vi "Voltage (with Events) - Continuous Input.vi"() -> ()   [LabVIEW 2022 SP3]
doc: "This example demonstrates how to continuously acquire buffered voltage measurements using a DAQmx device. It uses software events to ensure that the program does not become unresponsive while waiting for samples to become available.\n\nFor instructions on how to connect your signals to the DAQ device, refer to your device documentation."
uses:
  <vilib>/Utility/error.llb/DialogType.ctl
  <vilib>/DAQmx/read.llb/DAQmx Read (Analog 1D Wfm NChan NSamp).vi
  <vilib>/DAQmx/create/channels.llb/DAQmx Create Channel (AI-Voltage-Basic).vi
  <vilib>/DAQmx/configure/timing.llb/DAQmx Timing (Sample Clock).vi
  <vilib>/DAQmx/configure/task.llb/DAQmx Configure Logging (TDMS).vi
  <vilib>/DAQmx/configure/trigger.llb/DAQmx Start Trigger (Digital Edge).vi
  <vilib>/DAQmx/configure/trigger.llb/DAQmx Start Trigger (Time).vi
  <vilib>/DAQmx/configure/trigger.llb/DAQmx Start Trigger (Analog Edge).vi
  <vilib>/DAQmx/miscellaneous.llb/DAQmx Fill In Error Info.vi
  <resource>/objmgr/daqmx.rc
panel:
  in  "Trigger Type":T1(tab)
  in  "Digital Start Trigger Edge":i32(ring)=10280 caption="Edge" items=["Rising"=10280, "Falling"=10171]
  in  "Digital Start Trigger Source":tag="/Dev1/PFI0" caption="Source"
  in  "Digital Pause Trigger Pause When":i32(ring)=10192 caption="Pause When" items=["High"=10192, "Low"=10214]
  in  "Digital Pause Trigger Source":tag="/Dev1/PFI0" caption="Source"
  in  "Analog Start Trigger Level":dbl caption="Level" format="%0.2f"
  in  "Analog Start Trigger Hysteresis":dbl caption="Hysteresis" format="%.2f"
  in  "Analog Start Trigger Slope":i32(ring)=10280 caption="Slope" items=["Rising"=10280, "Falling"=10171]
  in  "Analog Start Trigger Source":string="APFI0" caption="Source"
  in  "Analog Pause Trigger Source":string="APFI0" caption="Source"
  in  "Analog Pause Trigger Pause When":i32(ring)=10093 caption="Pause When" items=["Above Level"=10093, "Below Level"=10107]
  in  "Analog Pause Trigger Level":dbl caption="Level" format="%.2f"
  in  "When":timestamp
  in  "Select Time\nManually":bool
  in  "Stop":bool
  out "Waveform Graph":waveform(dbl)[](graph)
  in  "TDMS File Path":path
  in  "Samples per Loop":i32=100
  in  "Sample Rate":dbl=1000.0
  in  "Sample Clock Source":tag="OnboardClock"
  in  "Terminal Configuration":i32(ring)=-1 items=["default"=-1, "RSE"=10083, "NRSE"=10078, "Differential"=10106, "Pseudodifferential"=12529]
  in  "Max Voltage":dbl=5.0
  in  "Min Voltage":dbl=-5.0
  in  "Physical Channel":tag="Dev1/ai0"
  out "Actual Sample Rate":dbl format="%0.2f"
  in  "Logging Mode":i32(ring)=10231 items=["Off"=10231, "Log and Read"=15842]
  # "Channel Settings"
  # "Acquired Data"
  # "Timing Settings"
  # "Trigger Settings"
  # "Logging Settings"
  # "To enable triggers, select a tab above, and configure the settings.\n\nNot all hardware supports all trigger types. Refer to your device documentation for more information."
  # "This trigger type is not supported in continuous sample timing. \n\nRefer to your device documentation for more information on which triggers are supported."
  # "This trigger type is not supported in continuous sample timing. \n\nRefer to your device documentation for more information on which triggers are supported."
  # "If time is not manually set, task will begin after 10 seconds"
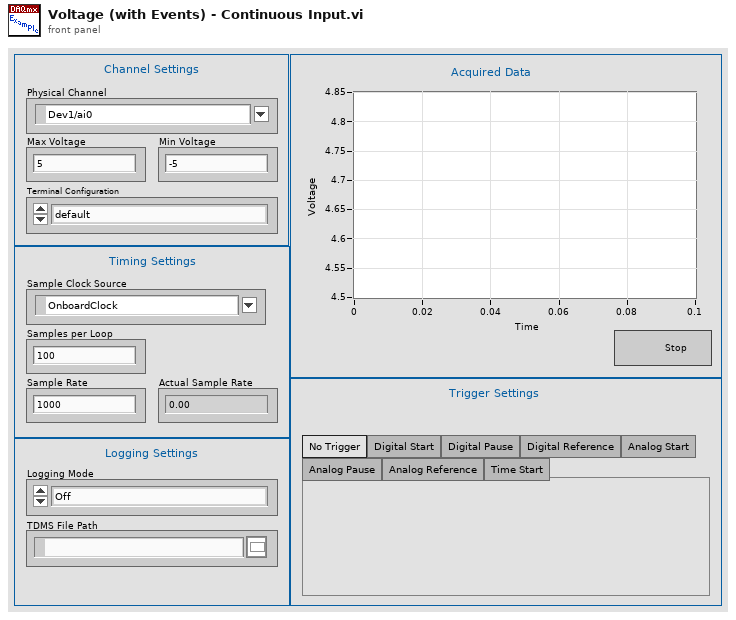
[diagram p1: front panel]
types:
  T1 = enum32{"No Trigger", "Digital Start", "Digital Pause", "Digital Reference", "Analog Start", "Analog Pause", "Analog Reference", "Time Start"}
  T2 = typedef "DialogType.ctl" = u16
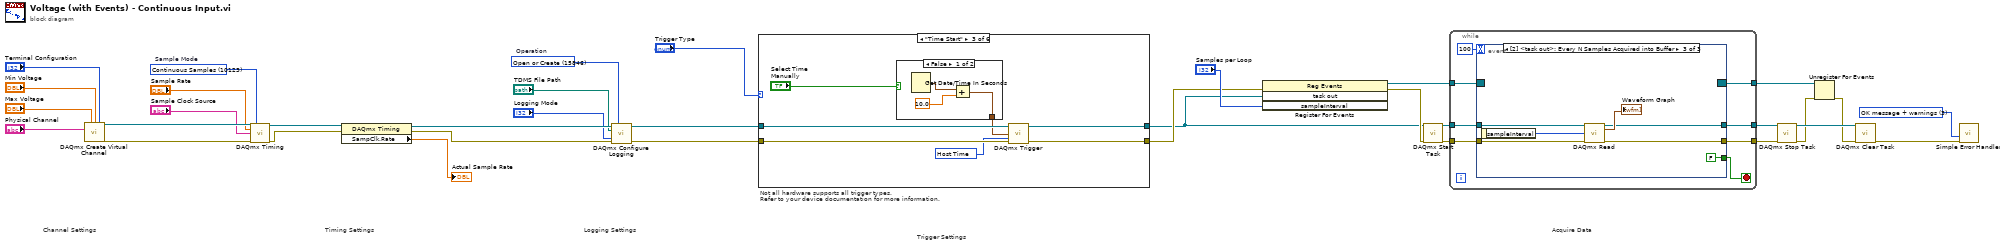
[diagram p0: block diagram]
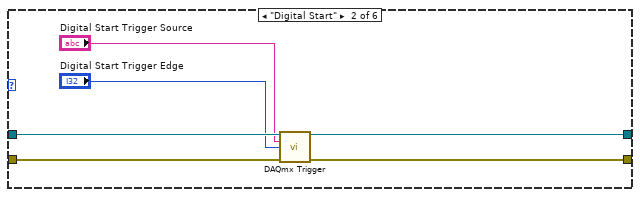
[diagram p3: hidden frame]
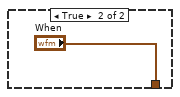
[diagram p4: hidden frame]
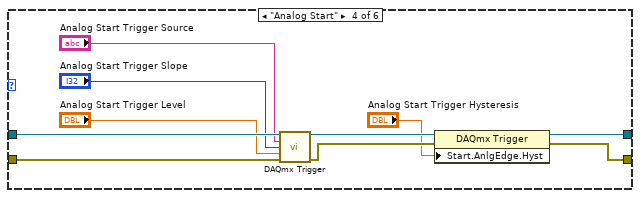
[diagram p5: hidden frame]
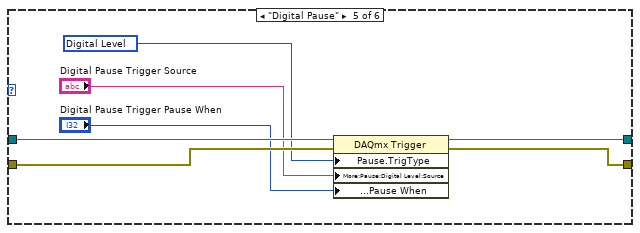
[diagram p6: hidden frame]
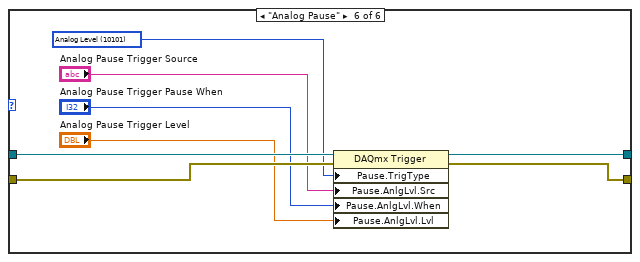
[diagram p7: hidden frame]
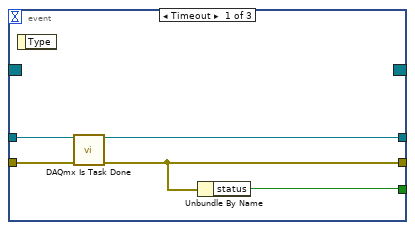
[diagram p8: hidden frame]
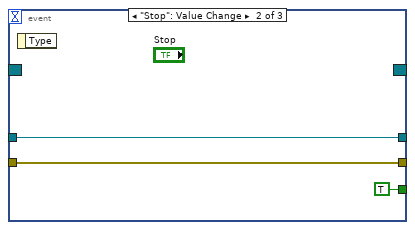
[diagram p9: hidden frame]
diagram:
  w9 = T2 3 items=["no dialog", "OK message", "continue or stop message", "OK message + warnings", "continue/stop + warnings"] ("type of dialog (OK msg:1)")
  w28 = 15846 items=["Open"=10437, "Open or Create"=15846, "Create or Replace"=15847, "Create"=15848]  # Operation
  w33 = 10123 items=["Finite Samples"=10178, "Continuous Samples"=10123, "Hardware Timed Single Point"=12522]  # Sample Mode
  # "Trigger Settings"
  # "Not all hardware supports all trigger types.\nRefer to your device documentation for more information."
  # "Acquire Data"
  # "Logging Settings"
  # "Timing Settings"
  # "Channel Settings"
  n1 = call-poly <vilib>:"DAQmx Create Virtual Channel.vi"("maximum value"="Max Voltage", "minimum value"="Min Voltage", "input terminal configuration"="Terminal Configuration", "physical channels"="Physical Channel") -> ("task out"=w31:refnum<k21>, "error out"=w32:errorcluster)  [unwired: 10 in]
  n2 = call-poly <vilib>:"DAQmx Timing.vi"("task/channels in"=w31, "sample mode"=w33, "rate"="Sample Rate", "source"="Sample Clock Source", "error in"=w32) -> ("task out"=w35:refnum<k21>, "error out"=w34:errorcluster)  [unwired: 9 in]
  n3 = property class="DAQmx Timing"(reference=w35, error in=w34) -> (reference out=w30:refnum<k21>, error out=w29:errorcluster, "SampClk.Rate"=→"Actual Sample Rate":dbl)
  n4 = call-poly <vilib>:"DAQmx Configure Logging.vi"("task/channels in"=w30, "operation"=w28, "file path"="TDMS File Path", "logging mode"="Logging Mode", "error in"=w29) -> ("task out"=w2:refnum<k21>, "error out"=w1:errorcluster)  [unwired: 9 in]
  n5 = case shown="\"Time Start\"" "Trigger Type" {
    tunnel: w2 -> [w37 w43 w50 w64 w71 w79]
    tunnel: w1 -> [w36 w42 w49 w63 w68 w76]
    tunnel: [w37 w41 w48 w61 w70 w78] -> w3
    tunnel: [w36 w40 w47 w60 w69 w77] -> w4
    frame "No Trigger", Default {
    }
    frame "Digital Start" {
      n6 = call-poly <vilib>:"DAQmx Trigger.vi"("task/channels in"=w43, "source"="Digital Start Trigger Source", "edge"="Digital Start Trigger Edge", "error in"=w42) -> ("task out"=w41:refnum<k21>, "error out"=w40:errorcluster)  [unwired: 10 in]
    }
    frame "Time Start" {
      w46 = 16126 items=["Host Time"=16126, "I/O Device Time"=16127] ("timescale")
      n7 = case shown="False" "Select Time\nManually" {
        tunnel: [w52 "When"] -> w44
        frame False {
          n8 = Get Date/Time In Seconds() -> (seconds since 1Jan1904=w53:timestamp)
          n9 = Add(x=w53, y=10.0) -> (x+y=w52:timestamp)
        }
        frame True {
        }
      }
      n10 = call-poly <vilib>:"DAQmx Trigger.vi"("task/channels in"=w50, "when"=w44, "timescale"=w46, "error in"=w49) -> ("task out"=w48:refnum<k21>, "error out"=w47:errorcluster)  [unwired: 10 in]
    }
    frame "Analog Start" {
      n11 = call-poly <vilib>:"DAQmx Trigger.vi"("task/channels in"=w64, "source"="Analog Start Trigger Source", "slope"="Analog Start Trigger Slope", "level"="Analog Start Trigger Level", "error in"=w63) -> ("task out"=w59:refnum<k21>, "error out"=w58:errorcluster)  [unwired: 9 in]
      n12 = property class="DAQmx Trigger"(reference=w59, error in=w58, "Start.AnlgEdge.Hyst"="Analog Start Trigger Hysteresis") -> (reference out=w61:refnum<k21>, error out=w60:errorcluster)
    }
    frame "Digital Pause" {
      w67 = 10152 items=["Analog Level"=10101, "Analog Window"=10103, "Digital Level"=10152, "Digital Pattern"=10398, "None"=10230] ("Pause.TrigType")
      n13 = property class="DAQmx Trigger"(reference=w71, error in=w68, "Pause.TrigType"=w67, "More:Pause:Digital Level:Source"="Digital Pause Trigger Source", "More:Pause:Digital Level:Pause When"="Digital Pause Trigger Pause When") -> (reference out=w70:refnum<k21>, error out=w69:errorcluster)
    }
    frame "Analog Pause" {
      w75 = 10101 items=["Analog Level"=10101, "Analog Window"=10103, "Digital Level"=10152, "Digital Pattern"=10398, "None"=10230] ("Pause.TrigType")
      n14 = property class="DAQmx Trigger"(reference=w79, error in=w76, "Pause.TrigType"=w75, "Pause.AnlgLvl.Src"="Analog Pause Trigger Source", "Pause.AnlgLvl.When"="Analog Pause Trigger Pause When", "Pause.AnlgLvl.Lvl"="Analog Pause Trigger Level") -> (reference out=w78:refnum<k21>, error out=w77:errorcluster)
    }
  }
  n15 = register-events(error in=w4, w3, "Samples per Loop") -> (reference out=w17:refnum<event-registration>, error out=w15:errorcluster)  [unwired: 1 in]
  n16 = call <vilib>:"DAQmx Start Task.vi"("task/channels in"=w3, "error in"=w15) -> ("task out"=w13:refnum<k21>, "error out"=w14:errorcluster)  [unwired: 12 in]
  n17 = while {
    tunnel: w17 -> [w87]
    tunnel: w14 -> [w86]
    tunnel: w13 -> [w85]
    tunnel: [w84] -> w10
    tunnel: [w83] -> w12
    tunnel: [w82] -> w8
    stop <- w81 stop-if-true
    n18 = event shown="[2] <task out>: Every N Samples Acquired into Buffer" {
      selector: w87 -> [_ _ _]
      dyn-events: [_ _ _] -> w83
      timeout: 100 ("Event Timeout") -> [_ _ _]
      tunnel: w86 -> [w91 w94 w100]
      tunnel: w85 -> [w92 w95 w101]
      tunnel: [w90 w95 w98] -> w84
      tunnel: [w89 w94 w97] -> w82
      tunnel: [w88 TRUE FALSE] -> w81
      event Timeout {
        n19 = event-data() -> ()  [unwired: 1 in, 1 out]
        n20 = call <vilib>:"DAQmx Is Task Done.vi"("task/channels in"=w92, "error in"=w91) -> ("task out"=w90:refnum<k21>, "error out"=w89:errorcluster)  [unwired: 11 in, 1 out]
        n21 = Unbundle By Name(w89) -> ("status"=w88:bool)
      }
      event "Stop": Value Change {
        n22 = event-data() -> ()  [unwired: 1 in, 1 out]
      }
      event Every N Samples Acquired into Buffer {
        n23 = event-data() -> ("sampleInterval"=w99:u32)  [unwired: 1 in]
        n24 = call-poly <vilib>:"DAQmx Read.vi"("task/channels in"=w101, "number of samples per channel"=w99, "error in"=w100) -> ("task out"=w98:refnum<k21>, "data"=→"Waveform Graph":waveform(dbl)[], "error out"=w97:errorcluster)  [unwired: 10 in]
      }
    }
  }
  n25 = call <vilib>:"DAQmx Stop Task.vi"("task/channels in"=w10, "error in"=w8) -> ("task out"=w11:refnum<k21>, "error out"=w7:errorcluster)  [unwired: 12 in]
  n26 = Unregister For Events(event registration refnum=w12, error in=w7) -> (error out=w6:errorcluster)
  n27 = call <vilib>:"DAQmx Clear Task.vi"("task in"=w11, "error in"=w6) -> ("error out"=w27:errorcluster)  [unwired: 13 in]
  n28 = call <vilib>:"Simple Error Handler.vi"("type of dialog (OK msg:1)"=w9, "error in (no error)"=w27) -> ()  [unwired: 3 in, 5 out]
